vi "Check wether Click is in Plot Area.vi"(8 "Error In":errorcluster, 9 "Mouse Click Coordinates":T2, 11 "Plot Bounds":T1) -> (0 "Error Out":errorcluster, 3 "Is in Plot Area?":bool)   [LabVIEW 2021, in "Graphs.lvlib"]
doc: "Determines whether the <b>Mouse Click Coordinates</b> are within the <b>Plot Bounds</b>."
uses:
  Graphs.lvlib
  <vilib>/Utility/miscctls.llb/LVPoint32TypeDef.ctl
  <vilib>/Utility/miscctls.llb/LVRectTypeDef.ctl
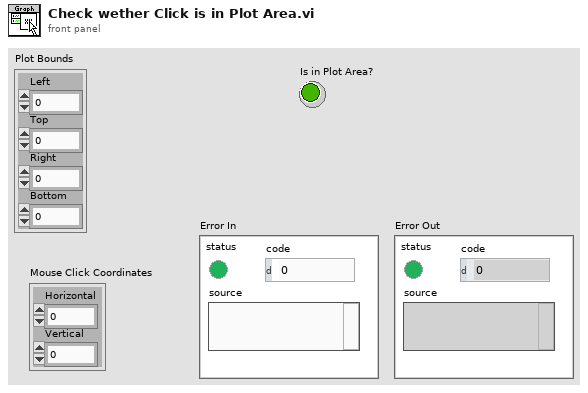
[diagram p1: front panel]
types:
  T1 = typedef "LVRectTypeDef.ctl" = cluster{"Left":i16, "Top":i16, "Right":i16, "Bottom":i16}
  T2 = typedef "LVPoint32TypeDef.ctl" = cluster{"Horizontal":i32, "Vertical":i32}
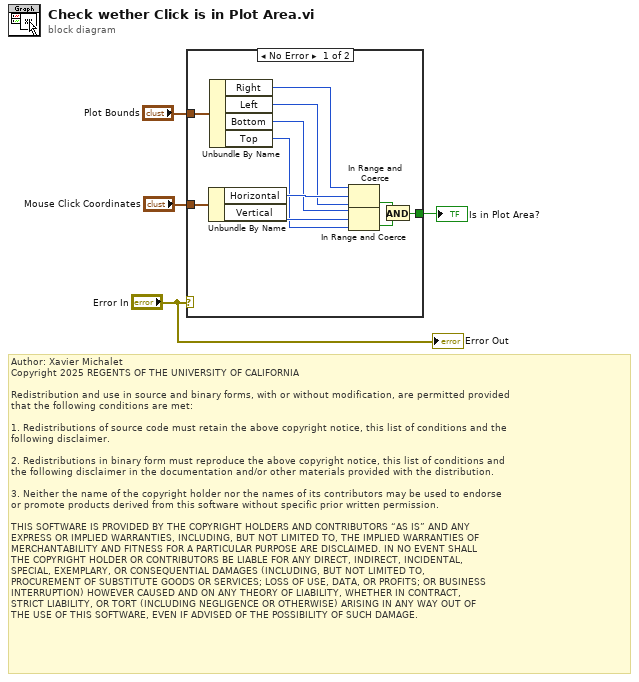
[diagram p0: block diagram]
diagram:
  # "Author: Xavier Michalet\nCopyright 2025 REGENTS OF THE UNIVERSITY OF CALIFORNIA\n\nRedistribution and use in source and binary forms, with or without modification, are permitted provided\nthat the following conditions are met:\n\n1. Redistributions of source code must retain the above copyright notice, this list of conditions and the\nfollowing disclaimer.\n\n2. Redistributions in binary form must reproduce the above copyright notice, this list of conditions and\nthe following disclaimer in the documentation and/or other materials provided with the distribution.\n\n3. Neither the name of the copyright holder nor the names of its contributors may be used to endorse \nor promote products derived from this software without specific prior written permission.\n\nTHIS SOFTWARE IS PROVIDED BY THE COPYRIGHT HOLDERS AND CONTRIBUTORS “AS IS” AND ANY \nEXPRESS OR IMPLIED WARRANTIES, INCLUDING, BUT NOT LIMITED TO, THE IMPLIED WARRANTIES OF\nMERCHANTABILITY AND FITNESS FOR A PARTICULAR PURPOSE ARE DISCLAIMED. IN NO EVENT SHALL\nTHE COPYRIGHT HOLDER OR CONTRIBUTORS BE LIABLE FOR ANY DIRECT, INDIRECT, INCIDENTAL, \nSPECIAL, EXEMPLARY, OR CONSEQUENTIAL DAMAGES (INCLUDING, BUT NOT LIMITED TO, \nPROCUREMENT OF SUBSTITUTE GOODS OR SERVICES; LOSS OF USE, DATA, OR PROFITS; OR BUSINESS\nINTERRUPTION) HOWEVER CAUSED AND ON ANY THEORY OF LIABILITY, WHETHER IN CONTRACT, \nSTRICT LIABILITY, OR TORT (INCLUDING NEGLIGENCE OR OTHERWISE) ARISING IN ANY WAY OUT OF\nTHE USE OF THIS SOFTWARE, EVEN IF ADVISED OF THE POSSIBILITY OF SUCH DAMAGE."
  n1 = case shown="No Error" "Error In" {
    tunnel: "Plot Bounds" -> [w15 _]
    tunnel: "Mouse Click Coordinates" -> [w14 _]
    tunnel: [w5 _] -> w2
    frame No Error {
      n2 = Unbundle By Name(w14) -> ("Horizontal"=w13:i32, "Vertical"=w10:i32)
      n3 = Unbundle By Name(w15) -> ("Right"=w12:i16, "Left"=w11:i16, "Bottom"=w9:i16, "Top"=w8:i16)
      n4 = In Range and Coerce(upper limit=w12, x=w13, lower limit=w11) -> (In Range?=w7:bool)  [unwired: 1 out]
      n5 = In Range and Coerce(upper limit=w9, x=w10, lower limit=w8) -> (In Range?=w6:bool)  [unwired: 1 out]
      n6 = And(x=w7, y=w6) -> (x .and. y?=w5:bool)
    }
    frame Error {
    }
  }
  "Is in Plot Area?" <- w2
  "Error Out" <- "Error In"
